vi "Set MCL Column Widths.vi"(8 "Error In":errorcluster, 9 "Total Width (pixels)":u32, 10 "Column Widths (pixels)":u32[](array[numeric]), 11 "MCL Ref In":refnum<vi>) -> (0 "Error Out":errorcluster, 3 "MCL Ref Out":refnum<vi>)   [LabVIEW 2023, in "Error Manager.lvlib"]
uses:
  <vilib>/Utility/miscctls.llb/LVRowAndColumnTypeDef.ctl
  Error Manager.lvlib
panel:
  # "Input\nInputs to the VI"
  # "Development\nControls or indicators that are useful for development or testing, but which are not outputs of the VI."
  # "Output\nOutputs of the VI"
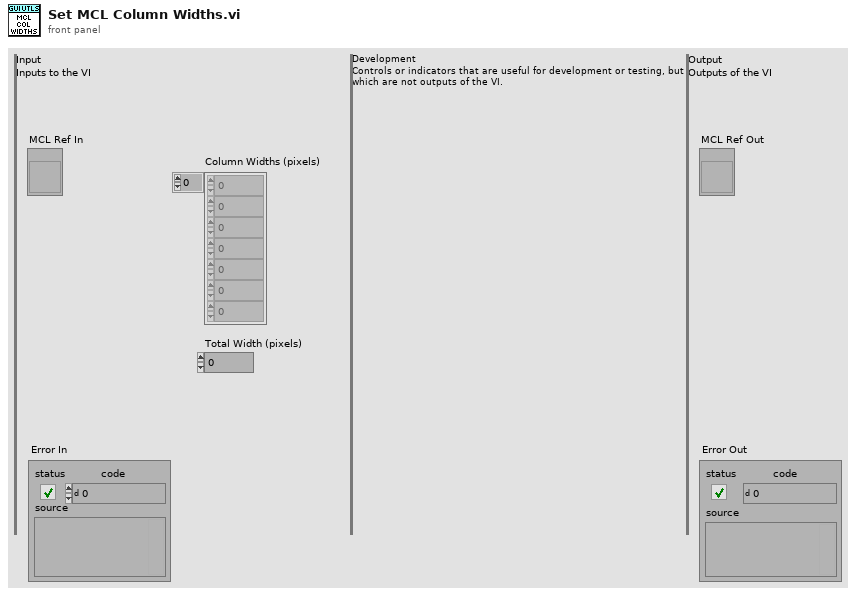
[diagram p1: front panel]
types:
  T1 = typedef "LVRowAndColumnTypeDef.ctl" = cluster{"Row":i32, "Column":i32}
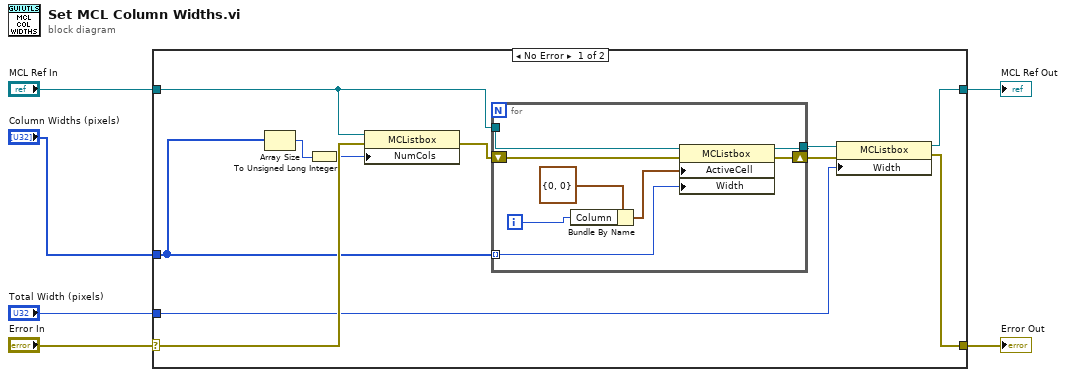
[diagram p0: block diagram]
diagram:
  n1 = case shown="No Error" "Error In" {
    selector: "Error In" -> [w15 w27]
    tunnel: [w12 w27] -> w5
    tunnel: "MCL Ref In" -> [w10 w26]
    tunnel: [w9 w26] -> w3
    tunnel: "Column Widths (pixels)" -> [w8 _]
    tunnel: "Total Width (pixels)" -> [w7 _]
    frame No Error {
      n2 = Array Size(array=w8) -> (size(s)=w16:i32)
      n3 = To Unsigned Long Integer(number=w16) -> (unsigned 32bit integer=w14:u32)
      n4 = property on="Property Node" class="MCListbox"(reference=w10, error in=w15, "NumCols"=w14) -> (error out=w17:errorcluster)  [unwired: 1 out]
      n5 = for {
        tunnel: w8 -> [w24] mode=indexing
        tunnel: w10 -> [w25]
        shift-right: [w20] -> w13
        shift-left: w17 -> [w19]
        tunnel: [w18] -> w11
        i -> [w22]
        n6 = Bundle By Name(cluster=T1 {"Row"=0, "Column"=0} ("Active Cell:Active Cell"), "Column"=w22) -> (w21:T1)
        n7 = property on="Property Node" class="MCListbox"(reference=w25, error in=w19, "ActiveCell"=w21, "Width"=w24) -> (reference out=w18:refnum<vi>, error out=w20:errorcluster)
      }
      n8 = property on="Property Node" class="MCListbox"(reference=w11, error in=w13, "Width"=w7) -> (reference out=w9:refnum<vi>, error out=w12:errorcluster)
    }
    frame Error {
    }
  }
  "Error Out" <- w5
  "MCL Ref Out" <- w3
